vi "Apply Low Pass Filter.vi"(8 "error in":errorcluster, 11 "4300 in":refnum<class "4300.lvclass">) -> (0 "error out":errorcluster, 3 "4300 out":refnum<class "4300.lvclass">)   [LabVIEW 2019, in "4300.lvlib" / "4300.lvclass"]
uses:
  Library/4300.lvclass
  C:/Users/Public/Documents/Development/builds/Instruments/AnalogInput.lvlibp/Library/AnalogInput.lvclass
  Library/4300.lvclass/4300.ctl
  builds/Instruments/AnalogInput.lvlibp/Accessors/GUI/Read Channel Names.vi
  builds/Instruments/AnalogInput.lvlibp/Accessors/Read Low Pass Filter.vi
  <resource>/objmgr/daqmx.rc
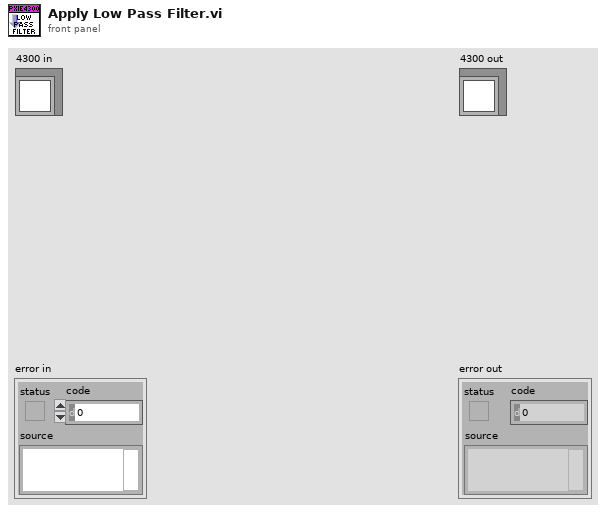
[diagram p1: front panel]
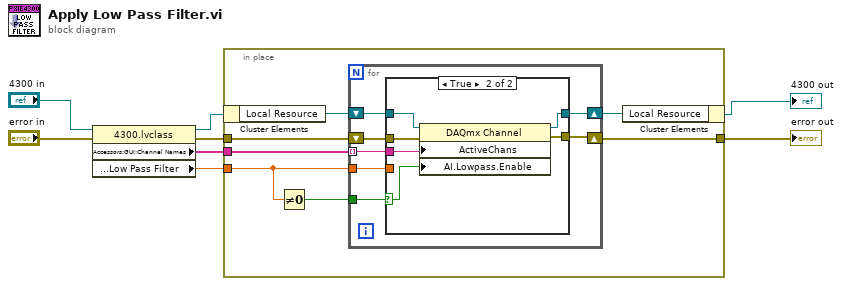
[diagram p0: block diagram]
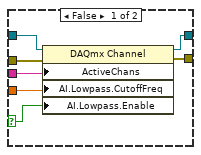
[diagram p2: hidden frame]
diagram:
  n1 = property class="4300.lvclass"(reference="4300 in", error in="error in") -> (reference out=w7:refnum<class "4300.lvclass">, error out=w2:errorcluster, "Accessors:GUI:Channel Names"=w4:string[], "Accessors:Config:Low Pass Filter"=w3:dbl)
  n2 = in-place {
    in-place-border: w4 -> [w11]
    in-place-border: w3 -> [w13]
    in-place-border: w2 -> [w10]
    in-place-border: [w9] -> w1
    n3 = in-place-cluster #1(w7) -> ("Local Resource"=w15:refnum<k21>)
    n4 = Not Equal To 0?(x=w13) -> (x != 0?=w12:bool)
    n5 = for {
      shift-right: [w20] -> w14
      shift-left: w15 -> [w21]
      tunnel: w13 -> [w16]
      tunnel: w12 -> [w17]
      tunnel: w11 -> [w22] mode=indexing
      shift-right: [w18] -> w9
      shift-left: w10 -> [w19]
      n6 = case shown="True" w17 {
        selector: w17 -> [w24 w30]
        tunnel: w22 -> [w29 w35]
        tunnel: w21 -> [w28 w34]
        tunnel: [w27 w33] -> w20
        tunnel: w19 -> [w26 w32]
        tunnel: [w25 w31] -> w18
        tunnel: w16 -> [w23 _]
        frame False {
          n7 = property class="DAQmx Channel"(reference=w28, error in=w26, "ActiveChans"=w29, "AI.Lowpass.CutoffFreq"=w23, "AI.Lowpass.Enable"=w24) -> (reference out=w27:refnum<k21>, error out=w25:errorcluster)
        }
        frame True {
          n8 = property class="DAQmx Channel"(reference=w34, error in=w32, "ActiveChans"=w35, "AI.Lowpass.Enable"=w30) -> (reference out=w33:refnum<k21>, error out=w31:errorcluster)
        }
      }
    }
    n9 = in-place-cluster #1("Local Resource"=w14) -> (→"4300 out":refnum<class "4300.lvclass">)
  }
  "error out" <- w1
